vi "Format Library Info Column.vi"(8 "error in (no error)":errorcluster {"code" format="Error %.0f"}, 9 "Column":T1, 10 "Library Info":T2, 11 "VIDoc Printer - Confluence In":refnum<class "VIDoc Printer - Confluence.lvclass">) -> (0 "error out":errorcluster {"code" format="Error %.0f"}, 1 "Header":string, 2 "Cell Text":string, 3 "VIDoc Printer - Confluence Out":refnum<class "VIDoc Printer - Confluence.lvclass">, 4 "Viable Value?":bool, 5 "Pixel Width":i16=275)   [LabVIEW 2023, in "VIDoc Printer - Confluence.lvlib" / "VIDoc Printer - Confluence.lvclass"]
uses:
  VIDoc Printer - Confluence.lvclass
  Parsing/TypeDefs/Base Library Info Cluster.ctl
  <vilib>/picture/picture.llb/imagedata.ctl
  Settings/Confluence Printer Settings/Class Info Column.ctl
  <userlib>/_PetranWay/LabVIEW Confluence API/Source/Confluence/HTML/Add Link to Text/Add URL to Text.vi
  VIDoc Printer - Confluence.lvclass/VIDoc Printer - Confluence.ctl
  Printer/VIDoc Printer.lvclass
  <userlib>/_PetranWay/LabVIEW Confluence API/Source/PetranWay_Confluence API.lvlib
  Settings/Confluence Printer Settings/VIDoc Settings - Confluence.lvclass
  Parsing/VIDoc Parsing.lvlib
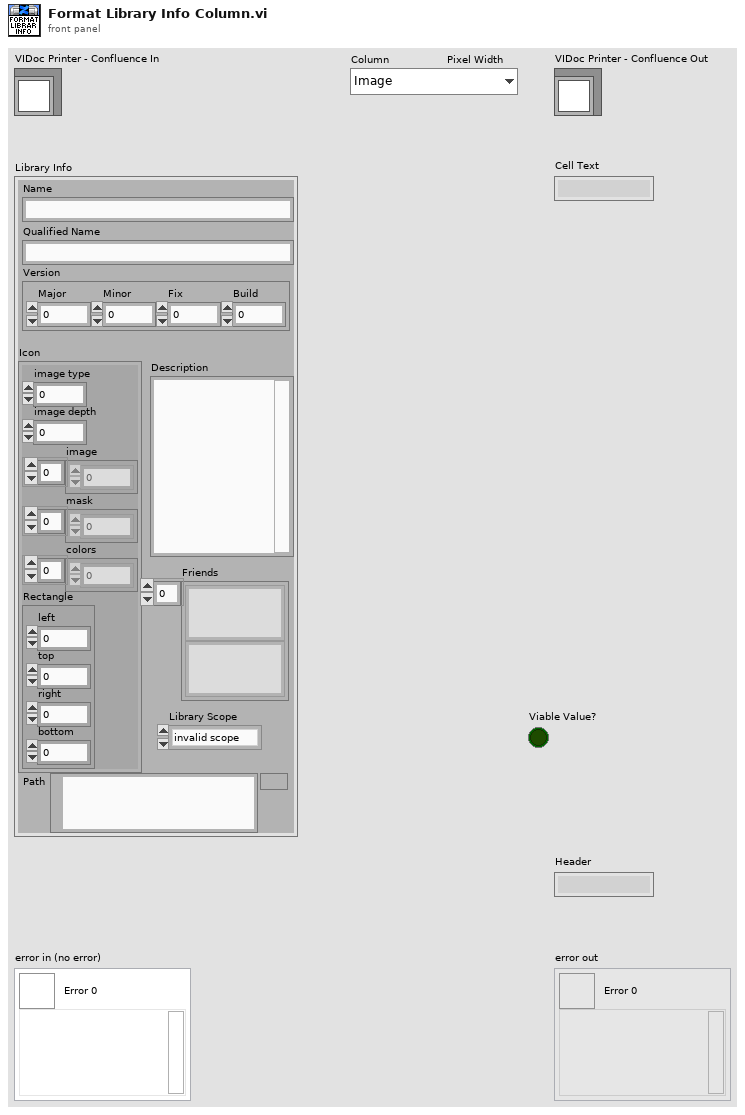
[diagram p1: front panel]
types:
  T1 = typedef "VIDoc Printer - Confluence.lvlib/VIDoc Settings - Confluence.lvclass/Class Info Column.ctl" = enum16{"Image", "Name", "Description", "Version", "Last Change", "Author", "Commit Hash", "Branch", "Qualified Name", "TransferMustOverrides", "ChildRefsRestricted"}
  T2 = typedef "VIDoc Parsing.lvlib/Base Library Info Cluster.ctl" = cluster{"Name":string, "Icon":T3, "Version":cluster{"Major":u16, "Minor":u16, "Fix":u16, "Build":u16}, "Description":string, "Path":path, "Friends":string[], "Library Scope":enum32{"invalid scope", "public", "private", "protected", "community"}, "Qualified Name":string}
  T3 = typedef "imagedata.ctl" = cluster{"image type":i32, "image depth":i32, "image":u8[], "mask":u8[], "colors":u32[], "Rectangle":cluster{"left":i16, "top":i16, "right":i16, "bottom":i16}}
  T4 = cluster{"Major":u16, "Minor":u16, "Fix":u16, "Build":u16}
  T5 = cluster{"Timestamp":timestamp, "Commit Hash":string, "Author Name":string, "Branch":string, "Commit Hash URL":string}
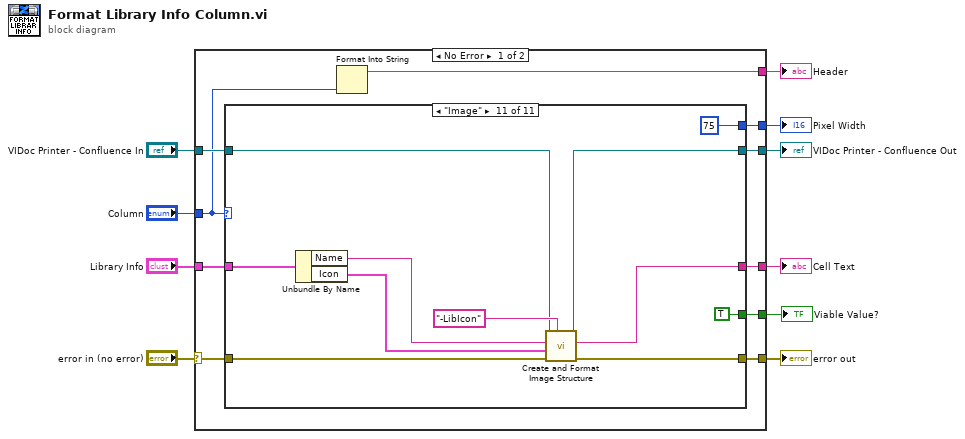
[diagram p0: block diagram]
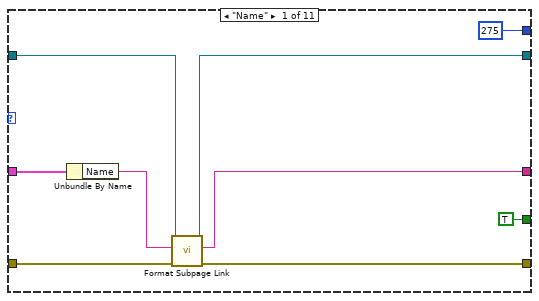
[diagram p2: hidden frame]
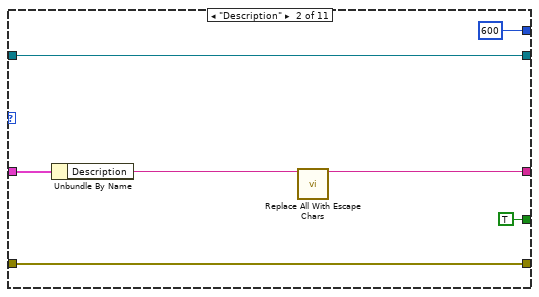
[diagram p3: hidden frame]
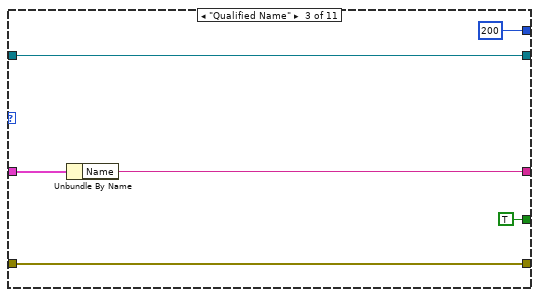
[diagram p4: hidden frame]
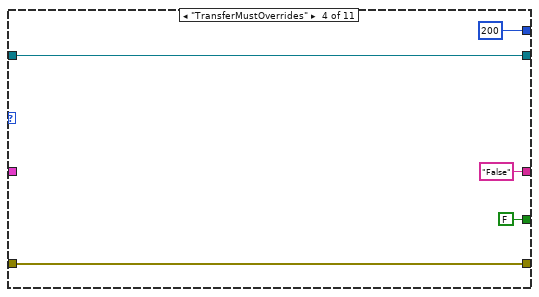
[diagram p5: hidden frame]
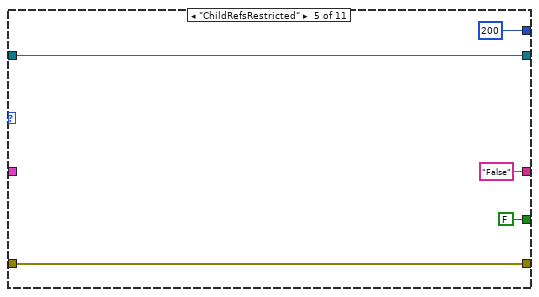
[diagram p6: hidden frame]
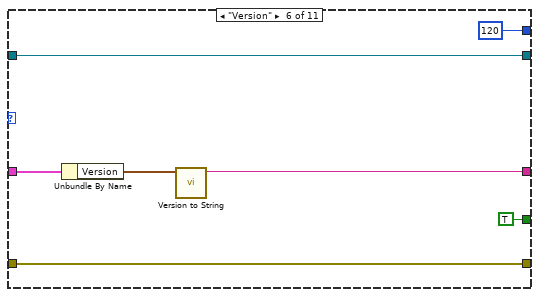
[diagram p7: hidden frame]
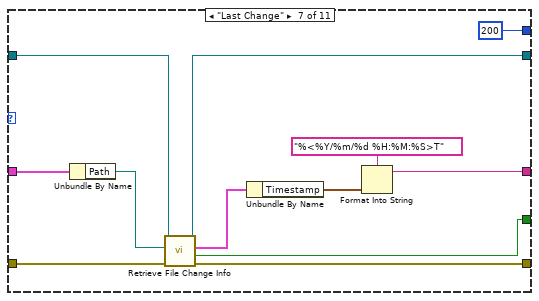
[diagram p8: hidden frame]
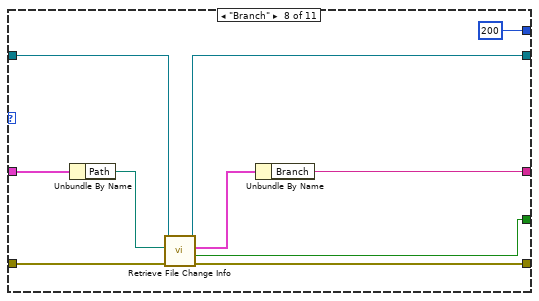
[diagram p9: hidden frame]
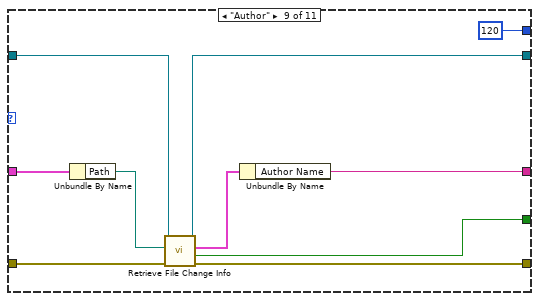
[diagram p10: hidden frame]
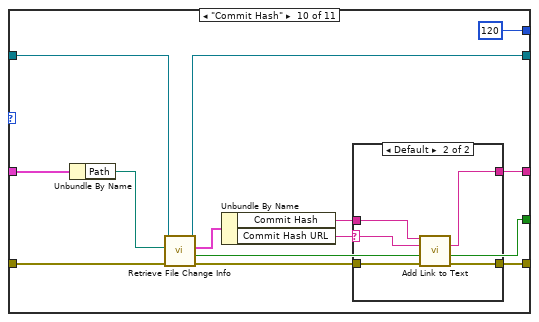
[diagram p11: hidden frame]
diagram:
  n1 = case shown="No Error" "error in (no error)" {
    selector: "error in (no error)" -> [w17 w124]
    tunnel: [w18 w124] -> w9
    tunnel: [w20 w123] -> w7
    tunnel: "VIDoc Printer - Confluence In" -> [w19 w123]
    tunnel: "Column" -> [w16 _]
    tunnel: [w15 _] -> w5
    tunnel: [w14 _] -> w4
    tunnel: "Library Info" -> [w13 _]
    tunnel: [w12 _] -> w2
    tunnel: [w11 _] -> w1
    frame No Error {
      n2 = case shown="\"Image\"" w16 {
        tunnel: [w25 w33 w39 w45 w50 w56 w63 w75 w85 w100 w116] -> w20
        tunnel: w19 -> [w24 w33 w39 w45 w50 w56 w62 w74 w84 w99 w117]
        tunnel: [w27 w34 w40 w46 w51 w57 w65 w77 w87 w95 w114] -> w18
        tunnel: w17 -> [w26 w34 w40 w46 w51 w57 w66 w78 w88 w102 w119]
        tunnel: [i16 275 ("Pixel Width") i16 600 ("Pixel Width") i16 200 ("Pixel Width") i16 200 ("Pixel Width") i16 200 ("Pixel Width") i16 120 ("Pixel Width") i16 200 ("Pixel Width") i16 200 ("Pixel Width") i16 120 ("Pixel Width") i16 120 ("Pixel Width") i16 75 ("Pixel Width")] -> w14
        tunnel: w13 -> [w28 w35 w41 _ _ w58 w70 w80 w90 w103 w120]
        tunnel: [w22 w30 w38 "False" ("Image Structure Text") "False" ("Image Structure Text") w54 w61 w73 w83 w92 w115] -> w12
        tunnel: [TRUE ("File Change Info Available?") TRUE ("File Change Info Available?") TRUE ("File Change Info Available?") FALSE ("File Change Info Available?") FALSE ("File Change Info Available?") TRUE ("File Change Info Available?") w60 w72 w82 w98 TRUE ("File Change Info Available?")] -> w11
        frame "Name" {
          n3 = Unbundle By Name(w28) -> ("Name"=w23:string)
          n4 = call "Format Subpage Link.vi"("error in (no error)"=w26, "Qualified Name"=w23, "VIDoc Printer - Confluence In"=w24) -> ("error out"=w27:errorcluster, "Linked HTML"=w22:string, "VIDoc Printer - Confluence Out"=w25:refnum<class "VIDoc Printer - Confluence.lvclass">)  [unwired: 6 in]
        }
        frame "Description" {
          n5 = Unbundle By Name(w35) -> ("Description"=w32:string)
          n6 = call <userlib>:"Replace All With Escape Chars.vi"("Raw String"=w32) -> ("With Substitued Escape Characters"=w30:string)  [unwired: 13 in, 1 out]
        }
        frame "Qualified Name" {
          n7 = Unbundle By Name(w41) -> ("Name"=w38:string)
        }
        frame "TransferMustOverrides" {
        }
        frame "ChildRefsRestricted" {
        }
        frame "Version" {
          n8 = Unbundle By Name(w58) -> ("Version"=w55:T4)
          n9 = call "Version to String.vi"("Version"=w55) -> ("String"=w54:string)  [unwired: 10 in]
        }
        frame "Last Change" {
          n10 = Unbundle By Name(w70) -> ("Path"=w64:path)
          n11 = call "Retrieve File Change Info.vi"("error in (no error)"=w66, "Absolute File Path"=w64, "VIDoc Printer - Confluence In"=w62) -> ("error out"=w65:errorcluster, "File Change Info Available?"=w60:bool, "File Change Info"=w69:T5, "VIDoc Printer - Confluence Out"=w63:refnum<class "VIDoc Printer - Confluence.lvclass">)  [unwired: 5 in]
          n12 = Unbundle By Name(w69) -> ("Timestamp"=w68:timestamp)
          n13 = Format Into String(format string="%<%Y/%m/%d %H:%M:%S>T", w68) -> (resulting string=w61:string)  [unwired: 2 in, 1 out]
        }
        frame "Branch" {
          n14 = Unbundle By Name(w80) -> ("Path"=w76:path)
          n15 = call "Retrieve File Change Info.vi"("error in (no error)"=w78, "Absolute File Path"=w76, "VIDoc Printer - Confluence In"=w74) -> ("error out"=w77:errorcluster, "File Change Info Available?"=w72:bool, "File Change Info"=w79:T5, "VIDoc Printer - Confluence Out"=w75:refnum<class "VIDoc Printer - Confluence.lvclass">)  [unwired: 5 in]
          n16 = Unbundle By Name(w79) -> ("Branch"=w73:string)
        }
        frame "Author" {
          n17 = Unbundle By Name(w90) -> ("Path"=w86:path)
          n18 = call "Retrieve File Change Info.vi"("error in (no error)"=w88, "Absolute File Path"=w86, "VIDoc Printer - Confluence In"=w84) -> ("error out"=w87:errorcluster, "File Change Info Available?"=w82:bool, "File Change Info"=w89:T5, "VIDoc Printer - Confluence Out"=w85:refnum<class "VIDoc Printer - Confluence.lvclass">)  [unwired: 5 in]
          n19 = Unbundle By Name(w89) -> ("Author Name"=w83:string)
        }
        frame "Commit Hash" {
          n20 = Unbundle By Name(w103) -> ("Path"=w101:path)
          n21 = call "Retrieve File Change Info.vi"("error in (no error)"=w102, "Absolute File Path"=w101, "VIDoc Printer - Confluence In"=w99) -> ("error out"=w93:errorcluster, "File Change Info Available?"=w98:bool, "File Change Info"=w94:T5, "VIDoc Printer - Confluence Out"=w100:refnum<class "VIDoc Printer - Confluence.lvclass">)  [unwired: 5 in]
          n22 = Unbundle By Name(w94) -> ("Commit Hash"=w97:string, "Commit Hash URL"=w96:string)
          n23 = case shown="Default" w96 {
            selector: w96 -> [_ w109]
            tunnel: w97 -> [w106 w111]
            tunnel: [w106 w110] -> w92
            tunnel: w93 -> [w105 w108]
            tunnel: [w105 w107] -> w95
            frame "" {
            }
            frame Default {
              n24 = call-poly <userlib>:"Add Link to Text.vi"("Text"=w111, "URL"=w109, "error in (no error)"=w108) -> ("HTML Text String"=w110:string, "error out"=w107:errorcluster)  [unwired: 10 in, 1 out]
            }
          }
        }
        frame "Image" {
          n25 = Unbundle By Name(w120) -> ("Name"=w112:string, "Icon"=w113:T3)
          n26 = call "Create and Format Image Structure.vi"("Name Addition"="-LibIcon" ("string"), "Error in"=w119, "Image Data"=w113, "Name"=w112, "VIDoc Printer - Confluence In"=w117) -> ("Error out"=w114:errorcluster, "Image Structure Text"=w115:string, "VIDoc Printer - Confluence Out"=w116:refnum<class "VIDoc Printer - Confluence.lvclass">)  [unwired: 3 in, 1 out]
        }
      }
      n27 = Format Into String(w16) -> (resulting string=w15:string)  [unwired: 3 in, 1 out]
    }
    frame Error {
    }
  }
  "error out" <- w9
  "VIDoc Printer - Confluence Out" <- w7
  "Pixel Width" <- w4
  "Cell Text" <- w2
  "Header" <- w5
  "Viable Value?" <- w1
